vi "test_libssh2_channel_direct_tcpip_ex.vi"() -> ()   [LabVIEW 2017, in "integration_tests.lvlib"]
uses:
  integration_tests.lvlib
  support/support.lvlib
  libssh2/libssh2.lvlib
  <vilib>/PNR/Transparent Assertions/Transparent Assertions/Transparent Assertions.lvlib
panel:
  out "error out":errorcluster
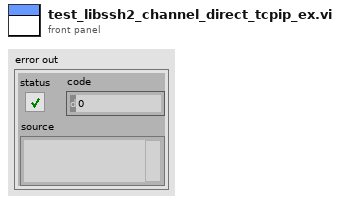
[diagram p1: front panel]
types:
  T1 = typedef "libssh2.lvlib/Session Refnum.ctl" = refnum<k1>
  T2 = typedef "libssh2.lvlib/Channel Refnum.ctl" = refnum<k1>
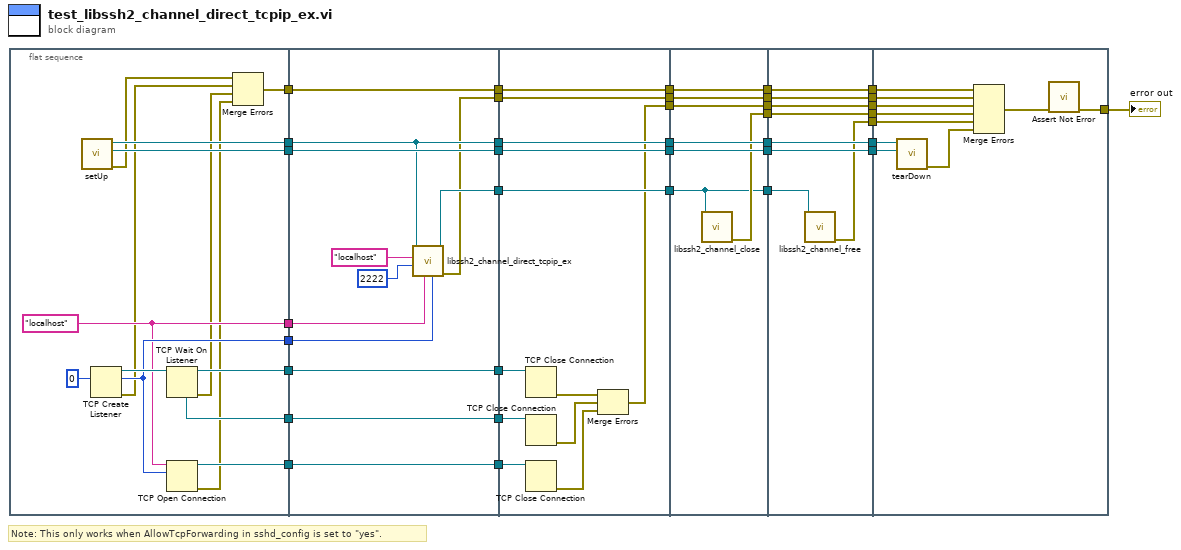
[diagram p0: block diagram]
diagram:
  # "Note: This only works when AllowTcpForwarding in sshd_config is set to \"yes\"."
  n1 = flat-sequence {
    tunnel: [w51] -> w37
    tunnel: [w50] -> w36
    tunnel: [w41] -> w35
    tunnel: [w47] -> w19
    tunnel: [w46] -> w18
    tunnel: [w45] -> w17
    tunnel: [w44] -> w16
    tunnel: [w43] -> w15
    tunnel: w37 -> [w62]
    tunnel: w36 -> [w63]
    tunnel: [w62] -> w34
    tunnel: [w63] -> w33
    tunnel: w35 -> [w61]
    tunnel: [w61] -> w32
    tunnel: [w60] -> w31
    tunnel: w19 -> [w57]
    tunnel: w18 -> [w56]
    tunnel: w17 -> [w54]
    tunnel: w16 -> [w53]
    tunnel: w15 -> [w55]
    tunnel: [w55] -> w14
    tunnel: [w54] -> w13
    tunnel: [w53] -> w12
    tunnel: [w52] -> w4
    tunnel: w34 -> [w75]
    tunnel: [w75] -> w9
    tunnel: w33 -> [w74]
    tunnel: [w74] -> w8
    tunnel: w32 -> [w73]
    tunnel: [w73] -> w7
    tunnel: w31 -> [w72]
    tunnel: [w72] -> w6
    tunnel: w14 -> [w71]
    tunnel: w13 -> [w70]
    tunnel: w12 -> [w69]
    tunnel: [w65] -> w5
    tunnel: w4 -> [w64]
    tunnel: [w64] -> w3
    tunnel: w9 -> [w82]
    tunnel: w8 -> [w81]
    tunnel: [w82] -> w30
    tunnel: [w81] -> w29
    tunnel: [w78] -> w28
    tunnel: [w80] -> w27
    tunnel: w7 -> [w79]
    tunnel: [w79] -> w26
    tunnel: w6 -> [w78]
    tunnel: [w77] -> w10
    tunnel: w5 -> [w77]
    tunnel: w3 -> [w76]
    tunnel: [w76] -> w2
    tunnel: w30 -> [w90]
    tunnel: w29 -> [w89]
    tunnel: w28 -> [w88]
    tunnel: [w90] -> w25
    tunnel: [w89] -> w24
    tunnel: [w87] -> w23
    tunnel: w27 -> [w86]
    tunnel: [w86] -> w22
    tunnel: w26 -> [w85]
    tunnel: [w85] -> w21
    tunnel: [w84] -> w11
    tunnel: w10 -> [w84]
    tunnel: w2 -> [w83]
    tunnel: [w83] -> w1
    tunnel: w25 -> [w100]
    tunnel: w24 -> [w99]
    tunnel: [w92] -> w20
    tunnel: w23 -> [w97]
    tunnel: w22 -> [w96]
    tunnel: w21 -> [w95]
    tunnel: w11 -> [w93]
    tunnel: w1 -> [w91]
    frame #0 {
      w46 = "localhost" ("shost")
      n2 = call "setUp.vi"() -> ("error out"=w42:errorcluster, "connection ID"=w50:refnum<k5>, "session"=w51:T1)  [unwired: 9 in]
      n3 = TCP Create Listener(10:u16 0 ("port")) -> (0:w40:errorcluster, 2:w47:u16, 3:w49:refnum<k5>)  [unwired: 4 in]
      n4 = TCP Wait On Listener(11:w49) -> (0:w39:errorcluster, 3:w43:refnum<k5>, 4:w45:refnum<k5>)  [unwired: 3 in, 2 out]
      n5 = TCP Open Connection(address=w46, remote port or service name=w47) -> (connection ID=w44:refnum<k5>, error out=w38:errorcluster)  [unwired: 3 in]
      n6 = Merge Errors(w42, w40, w39, w38) -> (w41:errorcluster)
    }
    frame #1 {
      n7 = call "libssh2_channel_direct_tcpip_ex.vi"("sport"=w57, "shost"=w56, "port"=2222, "host"="localhost", "session"=w62) -> ("error out"=w52:errorcluster, "channel"=w60:T2)  [unwired: 5 in]
    }
    frame #2 {
      n8 = TCP Close Connection(connection ID=w71) -> (error out=w68:errorcluster)  [unwired: 2 in, 1 out]
      n9 = TCP Close Connection(connection ID=w70) -> (error out=w67:errorcluster)  [unwired: 2 in, 1 out]
      n10 = TCP Close Connection(connection ID=w69) -> (error out=w66:errorcluster)  [unwired: 2 in, 1 out]
      n11 = Merge Errors(w68, w67, w66) -> (w65:errorcluster)
    }
    frame #3 {
      n12 = call "libssh2_channel_close.vi"("channel"=w78) -> ("error out"=w80:errorcluster)  [unwired: 10 in]
    }
    frame #4 {
      n13 = call "libssh2_channel_free.vi"("channel"=w88) -> ("error out"=w87:errorcluster)  [unwired: 10 in]
    }
    frame #5 {
      n14 = call "tearDown.vi"("connection ID"=w99, "session"=w100) -> ("error out"=w98:errorcluster)  [unwired: 9 in]
      n15 = Merge Errors(w95, w91, w93, w96, w97, w98) -> (w94:errorcluster)
      n16 = call <vilib>:"Assert Not Error.vi"("error in (no error)"=w94) -> ("error out"=w92:errorcluster)  [unwired: 10 in]
    }
  }
  "error out" <- w20
